vi "Airmar Init Sensor.vi"(8 "error in (no error)":errorcluster, 10 "NotifierReff":T1, 11 "VISA Refnum in":refnum<visa-resource-name>="COM1") -> (0 "error out":errorcluster, 2 "Try #":i32, 3 "VISA Refnum out":refnum<visa-resource-name>)   [LabVIEW 2013]
doc: "This VI checks to see if the sensor is communicating on 4800 or 38400 baud and sets it to 38400 baud if it is not already."
uses:
  Data/TypeDefs/Notifiers.ctl
  Data/TypeDefs/UTM Location.ctl
  Data/TypeDefs/Sail Set Suggestions.ctl
  Data/TypeDefs/Rudder Set Suggestions.ctl
  Data/TypeDefs/OverrideInformation.ctl
  Data/TypeDefs/OverrideMode.ctl
  Data/TypeDefs/MotorSetup.ctl
  Data/TypeDefs/DynamixelSetupInfo.ctl
  Data/TypeDefs/AirmarStatus.ctl
  Data/TypeDefs/HardwareOnline.ctl
  Data/TypeDefs/DynamixelCycleTracker.ctl
  Data/TypeDefs/RC Input Values.ctl
  Classes/Missions/GenericMission/GenericMission.lvclass
  Classes/Waypoint/Waypoint.lvclass
panel:
  out "# of serial connection attempts":i32
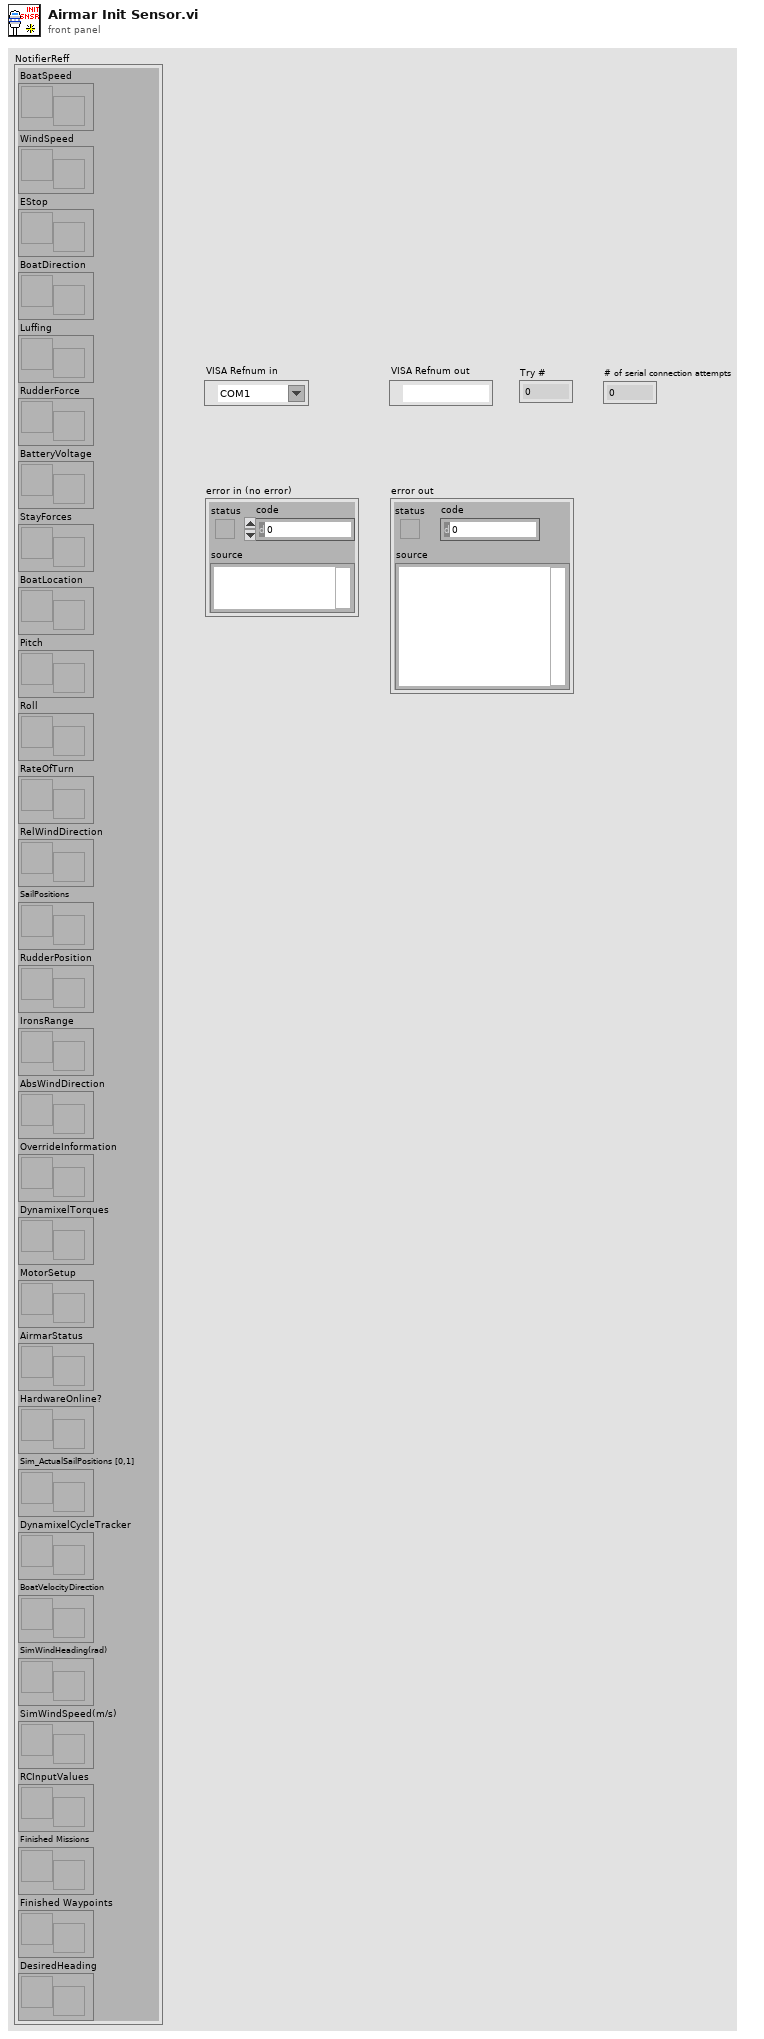
[diagram p1: front panel]
types:
  T1 = typedef "Notifiers.ctl" = cluster{"BoatSpeed":refnum<notifier>, "WindSpeed":refnum<notifier>, "EStop":refnum<notifier>, "BoatDirection":refnum<notifier>, "Luffing":refnum<notifier>, "RudderForce":refnum<notifier>, "BatteryVoltage":refnum<notifier>, "StayForces":refnum<notifier>, "BoatLocation":refnum<notifier>, "Pitch":refnum<notifier>, "Roll":refnum<notifier>, "RateOfTurn":refnum<notifier>, "RelWindDirection":refnum<notifier>, "SailPositions":refnum<notifier>, "RudderPosition":refnum<notifier>, "IronsRange":refnum<notifier>, "AbsWindDirection":refnum<notifier>, "OverrideInformation":refnum<notifier>, "DynamixelTorques":refnum<notifier>, "MotorSetup":refnum<notifier>, "AirmarStatus":refnum<notifier>, "HardwareOnline?":refnum<notifier>, "Sim_ActualSailPositions [0,1]":refnum<notifier>, "DynamixelCycleTracker":refnum<notifier>, "BoatVelocityDirection":refnum<notifier>, "SimWindHeading(rad)":refnum<notifier>, "SimWindSpeed(m/s)":refnum<notifier>, "RCInputValues":refnum<notifier>, "Finished Missions":refnum<notifier>, "Finished Waypoints":refnum<notifier>, "DesiredHeading":refnum<notifier>}
  T2 = typedef "HardwareOnline.ctl" = cluster{"AirmarOnline":bool, "WindvaneOnline":bool, "HemisphereOnline":bool, "StayForceOnline":bool, "BatteryVoltageOnline":bool, "AccelerometerOnline":bool, "MainDynamixel Online":bool, "JibDynamixel Online":bool, "RudderDynamixel Online":bool}
  T3 = typedef "AirmarStatus.ctl" = cluster{"Sensor Connected":bool, "Sensor Initialized":bool, "Sensor OK":bool, "Latest Error String":bool, "GPS Lock":bool}
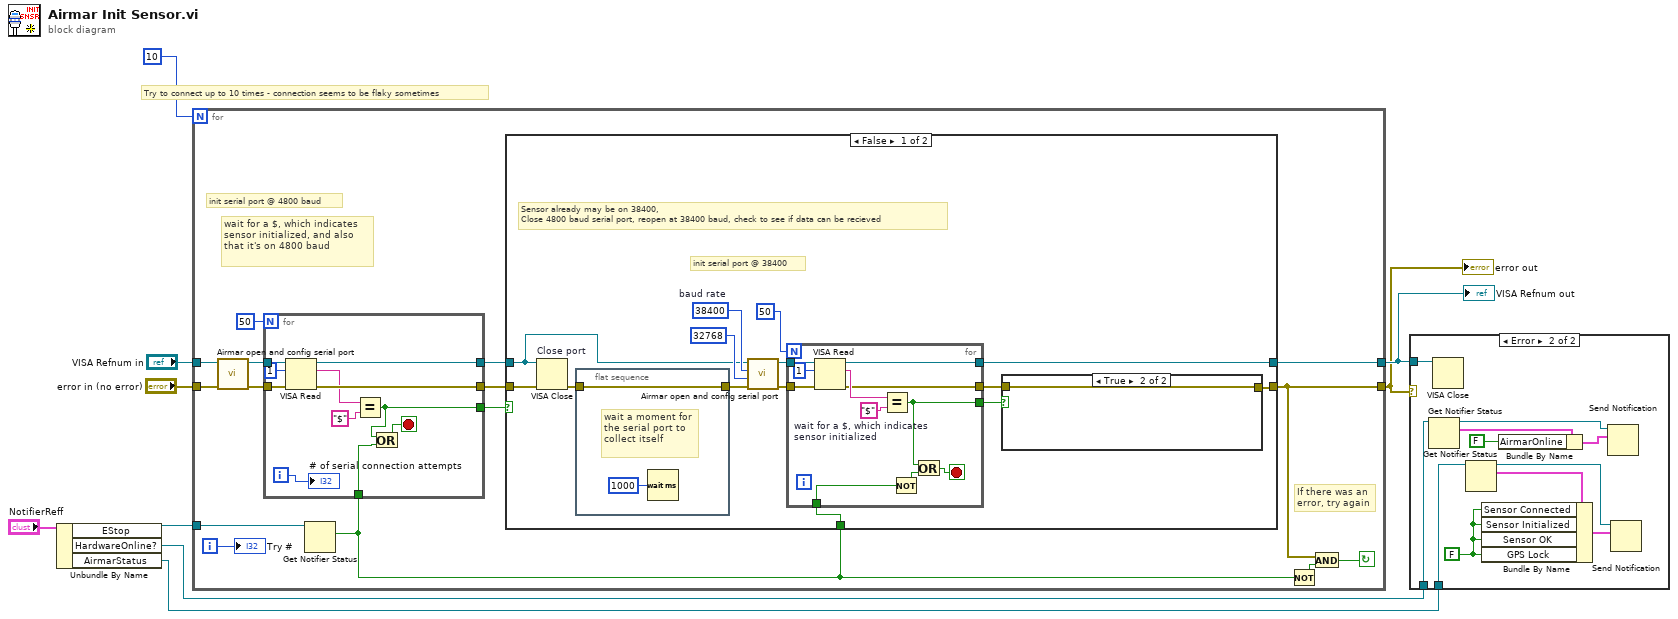
[diagram p0: block diagram]
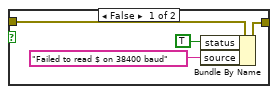
[diagram p2: hidden frame]
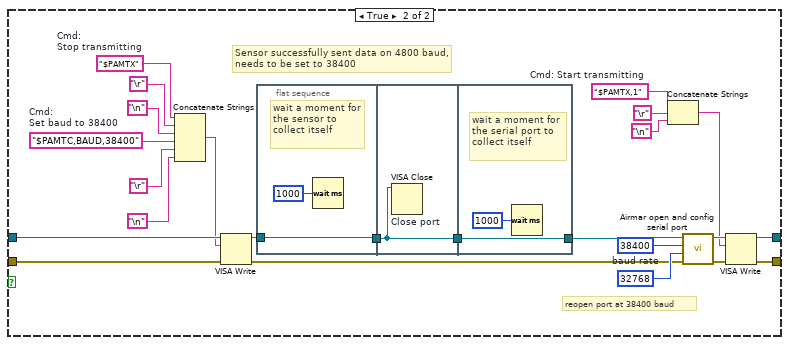
[diagram p3: hidden frame]
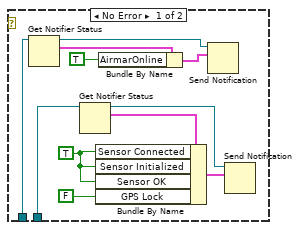
[diagram p4: hidden frame]
diagram:
  # "Try to connect up to 10 times - connection seems to be flaky sometimes"
  n1 = Unbundle By Name("NotifierReff") -> ("EStop"=w3:refnum<notifier>, "HardwareOnline?"=w2:refnum<notifier>, "AirmarStatus"=w1:refnum<notifier>)
  n2 = for {
    N: 10 -> [_]
    tunnel: "error in (no error)" -> [w24]
    tunnel: "VISA Refnum in" -> [w23]
    tunnel: [w22] -> w7
    tunnel: [w14] -> w6
    tunnel: w3 -> [w10]
    i -> [w16]
    stop <- w15 continue-if-true
    # "If there was an \nerror, try again"
    # "wait for a $, which indicates sensor initialized, and also that it's on 4800 baud"
    # "init serial port @ 4800 baud"
    n3 = call "Airmar open and config serial port.vi"("error in (no error)"=w24, "VISA Refnum in"=w23) -> ("error out"=w19:errorcluster, "VISA Refnum out"=w20:refnum<visa-resource-name>)  [unwired: 8 in]
    n4 = Get Notifier Status(notifier=w10) -> (current notification=w11:bool)  [unwired: 1 in, 4 out]
    n5 = for {
      N: 50 -> [_]
      tunnel: [w35] -> w21
      tunnel: w20 -> [w34]
      tunnel: w19 -> [w33]
      tunnel: [w32] -> w18
      tunnel: [w27] -> w17
      tunnel: w11 -> [w25]
      i -> [w26]
      stop <- w28 stop-if-true
      n6 = VISA Read(VISA resource name=w34, byte count=u32 1, error in (no error)=w33) -> (VISA resource name out=w35:refnum<visa-resource-name>, read buffer=w30:string, error out=w32:errorcluster)  [unwired: 1 out]
      n7 = Equal? ("wait for a $, which indicates\nsensor initialized")(x=w30, y="$" ("x")) -> (x = y?=w27:bool)
      n8 = Or(x=w27, y=w25) -> (x .or. y?=w28:bool)
      "# of serial connection attempts" <- w26
    }
    n9 = case shown="False" w17 {
      tunnel: [w45 w87] -> w22
      tunnel: w21 -> [w37 w79]
      tunnel: w18 -> [w40 w69]
      tunnel: [w44 w74] -> w14
      tunnel: w11 -> [w36 _]
      frame False {
        w49 = u32 38400  # baud rate
        # "init serial port @ 38400"
        # "Sensor already may be on 38400,\nClose 4800 baud serial port, reopen at 38400 baud, check to see if data can be recieved"
        n10 = VISA Close "Close port"(VISA resource name=w37, error in (no error)=w40) -> (error out=w39:errorcluster)
        n11 = flat-sequence {
          tunnel: w39 -> [w50]
          tunnel: [w50] -> w38
          frame #0 {
            # "wait a moment for the serial port to collect itself"
            n12 = Wait (ms)(milliseconds to wait=u32 1000) -> ()  [unwired: 1 out]
          }
        }
        n13 = call "Airmar open and config serial port.vi"("error in (no error)"=w38, "Input\nbuffer size"=u32 32768 ("Input\nbuffer size"), "baud rate"=w49, "VISA Refnum in"=w37) -> ("error out"=w46:errorcluster, "VISA Refnum out"=w47:refnum<visa-resource-name>)  [unwired: 6 in]
        n14 = for {
          N: 50 -> [_]
          tunnel: w47 -> [w62]
          tunnel: w46 -> [w61]
          tunnel: [w60] -> w45
          tunnel: [w53] -> w43
          tunnel: [w56] -> w42
          tunnel: w36 -> [w52]
          stop <- w54 stop-if-true
          n15 = VISA Read(VISA resource name=w62, byte count=u32 1, error in (no error)=w61) -> (VISA resource name out=w60:refnum<visa-resource-name>, read buffer=w58:string, error out=w56:errorcluster)  [unwired: 1 out]
          n16 = Equal? "wait for a $, which indicates\nsensor initialized"(x=w58, y="$" ("x")) -> (x = y?=w53:bool)
          n17 = Not(x=w52) -> (.not. x?=w55:bool)
          n18 = Or(x=w53, y=w55) -> (x .or. y?=w54:bool)
        }
        n19 = case shown="True" w43 {
          tunnel: w42 -> [w64 w67]
          tunnel: [w63 w67] -> w44
          frame False {
            n20 = Bundle By Name(cluster=w64, "status"=TRUE, "source"="Failed to read $ on 38400 baud") -> (w63:errorcluster)
          }
          frame True {
          }
        }
      }
      frame True {
        w73 = "$PAMTC,BAUD,38400"  # Cmd: Set baud to 38400
        w78 = "$PAMTX"  # Cmd: Stop transmitting
        w83 = "$PAMTX,1"  # Cmd: Start transmitting
        w89 = u32 38400  # baud rate
        # "Sensor successfully sent data on 4800 baud,\nneeds to be set to 38400"
        # "reopen port at 38400 baud"
        n21 = Concatenate Strings(w78, "\r" ("Carriage Return Constant"), "\n", w73, "\r" ("Carriage Return Constant"), "\n") -> (w77:string)
        n22 = VISA Write(VISA resource name=w79, write buffer=w77, error in (no error)=w69) -> (VISA resource name out=w70:refnum<visa-resource-name>, error out=w68:errorcluster)  [unwired: 1 out]
        n23 = flat-sequence {
          tunnel: w70 -> [w92]
          tunnel: [w92] -> w91
          tunnel: w91 -> [w94]
          tunnel: [w94] -> w90
          tunnel: [w96] -> w88
          tunnel: w90 -> [w96]
          frame #0 {
            # "wait a moment for the sensor to collect itself"
            n24 = Wait (ms)(milliseconds to wait=u32 1000) -> ()  [unwired: 1 out]
          }
          frame #1 {
            n25 = VISA Close "Close port"(VISA resource name=w94) -> ()  [unwired: 1 in, 1 out]
          }
          frame #2 {
            # "wait a moment for the serial port to collect itself"
            n26 = Wait (ms)(milliseconds to wait=u32 1000) -> ()  [unwired: 1 out]
          }
        }
        n27 = Concatenate Strings(w83, "\r" ("Carriage Return Constant"), "\n") -> (w80:string)
        n28 = call "Airmar open and config serial port.vi"("error in (no error)"=w68, "Input\nbuffer size"=u32 32768 ("Input\nbuffer size"), "baud rate"=w89, "VISA Refnum in"=w88) -> ("error out"=w86:errorcluster, "VISA Refnum out"=w84:refnum<visa-resource-name>)  [unwired: 6 in]
        n29 = VISA Write(VISA resource name=w84, write buffer=w80, error in (no error)=w86) -> (VISA resource name out=w87:refnum<visa-resource-name>, error out=w74:errorcluster)  [unwired: 1 out]
      }
    }
    n30 = Not(x=w11) -> (.not. x?=w13:bool)
    n31 = And(x=w14, y=w13) -> (x .and. y?=w15:bool)
    "Try #" <- w16
  }
  "VISA Refnum out" <- w7
  "error out" <- w6
  n32 = case shown="Error" w6 {
    tunnel: w7 -> [_ w118]
    tunnel: w2 -> [w103 w113]
    tunnel: w1 -> [w99 w112]
    frame No Error {
      w97 = TRUE
      n33 = Get Notifier Status(notifier=w103) -> (notifier out=w105:refnum<notifier>, current notification=w107:T2)  [unwired: 1 in, 3 out]
      n34 = Get Notifier Status(notifier=w99) -> (notifier out=w100:refnum<notifier>, current notification=w98:T3)  [unwired: 1 in, 3 out]
      n35 = Bundle By Name(cluster=w98, "Sensor Connected"=w97, "Sensor Initialized"=w97, "Sensor OK"=w97, "GPS Lock"=FALSE) -> (w101:T3)
      n36 = Bundle By Name(cluster=w107, "AirmarOnline"=TRUE) -> (w104:T2)
      n37 = Send Notification(notification=w104, notifier=w105) -> ()  [unwired: 1 in, 2 out]
      n38 = Send Notification(notification=w101, notifier=w100) -> ()  [unwired: 1 in, 2 out]
    }
    frame Error {
      w110 = FALSE ("GPS Lock")
      n39 = Get Notifier Status(notifier=w113) -> (notifier out=w115:refnum<notifier>, current notification=w117:T2)  [unwired: 1 in, 3 out]
      n40 = VISA Close(VISA resource name=w118) -> ()  [unwired: 1 in, 1 out]
      n41 = Get Notifier Status(notifier=w112) -> (notifier out=w109:refnum<notifier>, current notification=w111:T3)  [unwired: 1 in, 3 out]
      n42 = Bundle By Name(cluster=w111, "Sensor Connected"=w110, "Sensor Initialized"=w110, "Sensor OK"=w110, "GPS Lock"=w110) -> (w108:T3)
      n43 = Bundle By Name(cluster=w117, "AirmarOnline"=FALSE) -> (w114:T2)
      n44 = Send Notification(notification=w114, notifier=w115) -> ()  [unwired: 1 in, 2 out]
      n45 = Send Notification(notification=w108, notifier=w109) -> ()  [unwired: 1 in, 2 out]
    }
  }
